vi "Multi.vi"(0 "VisaCluster":T1, 7 "Multi":bool, 11 "error in (no error)":errorcluster) -> (4 "VisaCluster":T1, 8 "Answer":string, 15 "error out":errorcluster)   [LabVIEW 2014, in "FH 55.lvlib"]
doc: "This VI sets the Multi-Function ON or OFF.\n\nDurch dieses VI kann die automatische Messwertausgabe gestartet oder abgebrochen werden."
uses:
  FH 55.lvlib
  TypeDef/VisaCluster.ctl
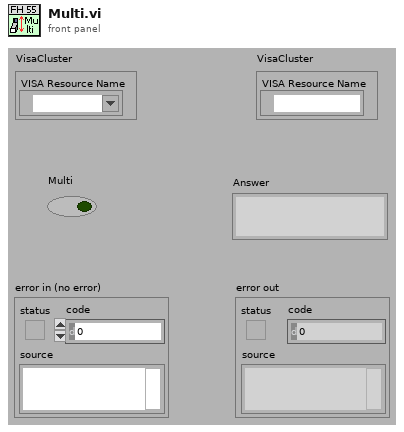
[diagram p1: front panel]
types:
  T1 = typedef "FH 55.lvlib/VisaCluster.ctl" = cluster{"VISA Resource Name":refnum<visa-resource-name>}
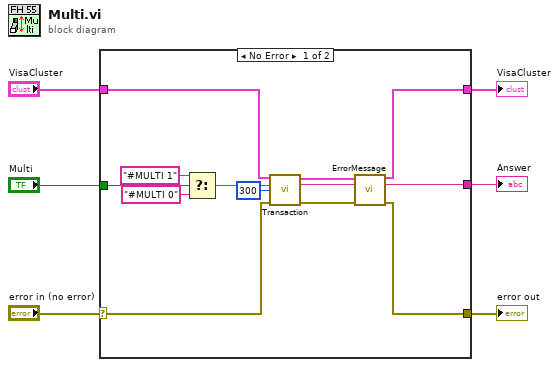
[diagram p0: block diagram]
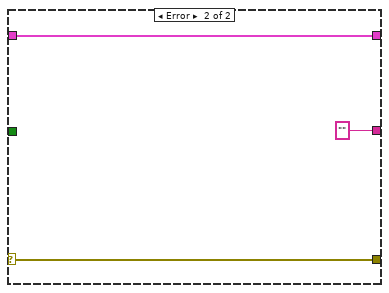
[diagram p2: hidden frame]
diagram:
  n1 = case shown="No Error" "error in (no error)" {
    selector: "error in (no error)" -> [w12 w21]
    tunnel: "VisaCluster" -> [w8 w22]
    tunnel: "Multi" -> [w19 _]
    tunnel: [w16 w22] -> w2
    tunnel: [w14 w21] -> w4
    tunnel: [w15 ""] -> w3
    frame No Error {
      n2 = Select(t="#MULTI 1", s=w19, f="#MULTI 0") -> (s? t:f=w13:string)
      n3 = call "Transaction.vi"("VisaCluster"=w8, "Command"=w13, "Time (150) ms"=u32 300, "error in (no error)"=w12) -> ("VisaCluster"=w9:T1, "Answer"=w10:string, "error out"=w11:errorcluster)  [unwired: 8 in, 1 out]
      n4 = call "ErrorMessage.vi"("VisaCluster"=w9, "Message In"=w10, "error in (no error)"=w11) -> ("VisaCluster"=w16:T1, "Message Out"=w15:string, "error out"=w14:errorcluster)  [unwired: 10 in]
    }
    frame Error {
    }
  }
  "error out" <- w4
  "Answer" <- w3
  "VisaCluster" <- w2
